vi "Timestamp to ISO8601 DateTime.vi"(9 "UTC? (F)":bool, 11 "Timestamp (now)":timestamp) -> (3 "ISO8601 DateTime":string)   [LabVIEW 2013]
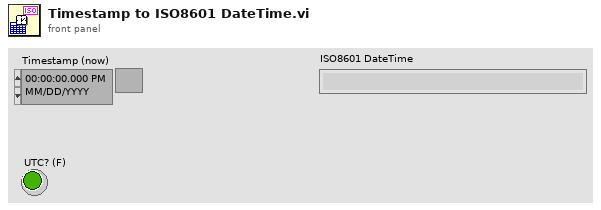
[diagram p1: front panel]
types:
  T1 = typedef "LVDateTimeRec.ctl" = cluster{"fractional second":dbl, "second":i32, "minute":i32, "hour":i32, "day of month":i32, "month":i32, "year":i32, "day of week":i32, "day of year":i32, "DST":i32}
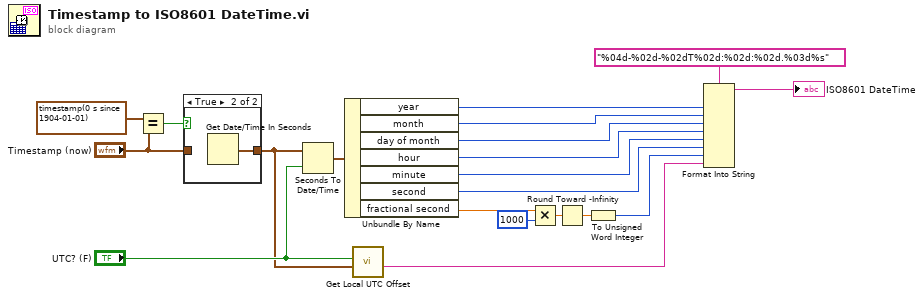
[diagram p0: block diagram]
diagram:
  n1 = Equal?(x=timestamp(0 s since 1904-01-01), y="Timestamp (now)") -> (x = y?=w3:bool)
  n2 = case shown="True" w3 {
    tunnel: [w21 w22] -> w1
    tunnel: "Timestamp (now)" -> [w21 _]
    frame False {
    }
    frame True {
      n3 = Get Date/Time In Seconds() -> (seconds since 1Jan1904=w22:timestamp)
    }
  }
  n4 = Seconds To Date/Time(time stamp (now)=w1, to UTC (F)="UTC? (F)") -> (date time rec=w17:T1)
  n5 = Unbundle By Name(w17) -> ("year"=w6:i32, "month"=w15:i32, "day of month"=w16:i32, "hour"=w14:i32, "minute"=w13:i32, "second"=w12:i32, "fractional second"=w10:dbl)
  n6 = call "Get Local UTC Offset.vi"("timestamp (now)"=w1, "UTC? (F)"="UTC? (F)") -> ("UTC Offset String"=w11:string)  [unwired: 8 in, 1 out]
  n7 = Multiply(x=w10, y=1000 ("upper limit")) -> (x*y=w8:dbl)
  n8 = Round Toward -Infinity(1:w8) -> (0:w5:dbl)
  n9 = To Unsigned Word Integer(number=w5) -> (unsigned 16bit integer=w7:u16)
  n10 = Format Into String(format string="%04d-%02d-%02dT%02d:%02d:%02d.%03d%s", w6, w15, w16, w14, w13, w12, w7, w11) -> (resulting string=→"ISO8601 DateTime":string)  [unwired: 2 in, 1 out]
